vi "Write Addr.vi"(8 "error in (no error)":errorcluster, 10 "Addr":refnum<visa-resource-name>, 11 "Lakeshore 336 in":refnum<class "Lakeshore 336.lvclass">) -> (0 "error out":errorcluster, 3 "Lakeshore 336 out":refnum<class "Lakeshore 336.lvclass">)   [LabVIEW 2022 SP3, in "Lakeshore 336.lvclass"]
uses:
  Lakeshore 336.lvclass
  Lakeshore 336.lvclass/Lakeshore 336.ctl
  Temp Control.lvclass
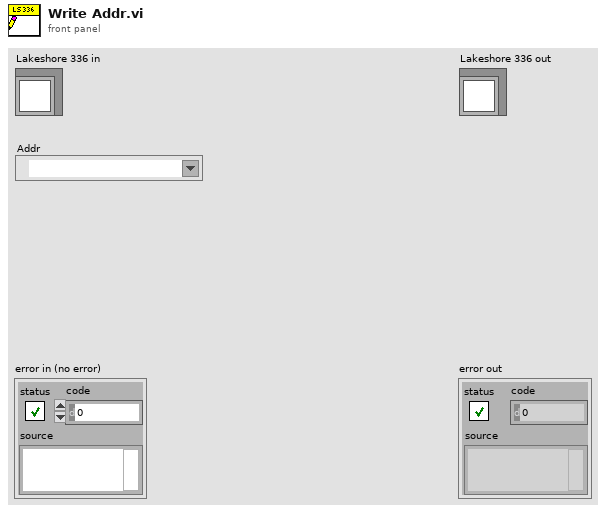
[diagram p1: front panel]
types:
  T1 = typedef "Lakeshore 336.lvclass/Lakeshore 336 Settings cluster.ctl" = cluster{"Lake Shore 336 Address":refnum<visa-resource-name>, "Output Ch":T2[], "Input Ch":T4[], "Prefix":string}
  T2 = typedef "Lakeshore 336.lvclass/Lakeshore 336 Channel Settings cluster.ctl" = cluster{"Input (0:None)":u16, "Power Up Enable (F: Off)":bool, "Mode (0:Off)":u16, "Max Current (0:User Specified)":u16, "Heater Out Display (1:Current)":u16, "Max User Current (2.000)":dbl, "Heater Resistance (1:25 Ohms)":u16, "PID":T3, "Name":string}
  T3 = typedef "Lakeshore 336.lvclass/Lakeshore 336 PID cluster.ctl" = cluster{"P":dbl, "I":dbl, "D":dbl}
  T4 = typedef "Lakeshore 336.lvclass/Lakeshore 336 Input Ch config cluster.ctl" = cluster{"Name":string}
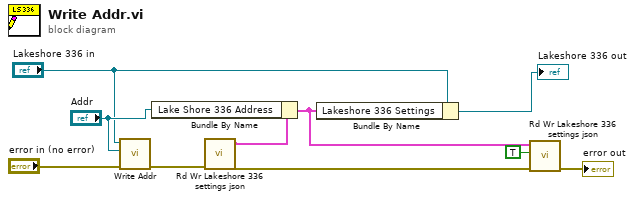
[diagram p0: block diagram]
diagram:
  n1 = call-parent "Write Addr.vi"("error in (no error)"="error in (no error)", "Addr"="Addr", "Temp Control in"="Lakeshore 336 in") -> ("error out"=w6:errorcluster)  [unwired: 7 in, 1 out]
  n2 = call "Rd Wr Lakeshore 336 settings json.vi"("error in (no error)"=w6) -> ("error out"=w1:errorcluster, "Lakeshore 336 Settings"=w5:T1)  [unwired: 9 in]
  n3 = Bundle By Name(cluster=w5, "Lake Shore 336 Address"="Addr") -> (w2:T1)
  n4 = Bundle By Name(cluster="Lakeshore 336 in", "Lakeshore 336 Settings"=w2) -> (→"Lakeshore 336 out":refnum<class "Lakeshore 336.lvclass">)
  n5 = call "Rd Wr Lakeshore 336 settings json.vi"("error in (no error)"=w1, "Write? (F:Read)"=TRUE, "Lakeshore 336 Settings"=w2) -> ("error out"=→"error out":errorcluster)  [unwired: 7 in, 1 out]
